vi "DPIDs.CompileServices.vi"(8 "error in (no error)":errorcluster, 11 "Section Ref in":T6 format="%.0x") -> (0 "error out":errorcluster, 1 "DPIDs Settings":T1[](array[typedef]), 2 "Settings":T3 {"Signal.Cmd.Refs"."Signal Refs" format="%.0x"; "Signal.Cmd.Info"."Signals"."Byte Order" items=["Little Endian", "Big Endian"]; "Signal.Cmd.Info"."Signals"."Data Type" items=["Signed", "Unsigned", "IEEE Float"]; "Settings.Refs"."Signal Refs" format="%.0x"; "Signal.Resp.Refs"."Signal Refs" format="%.0x"; "Signal.Resp.Info"."Signals"."Byte Order" items=["Little Endian", "Big Endian"]; "Signal.Resp.Info"."Signals"."Data Type" items=["Signed", "Unsigned", "IEEE Float"]; "Trigger.Refs"."Signal Refs" format="%.0x"; "Status.Refs"."Signal Refs" format="%.0x"}, 3 "Section Ref out":T6 format="%.0x")   [LabVIEW 2019, in "Diagnostics Addon System Explorer.lvlib"]
uses:
  Diagnostics Addon System Explorer.lvlib
  <vilib>/NI VeriStand/Custom Device API/Custom Device Item Ref.ctl
  Types/Service.Export.ctl
  Types/Frame.Ref.ctl
  Shared/Types/Type.ctl
  Shared/Types/Frame.Compile.ctl
  Shared/Types/Signal.ctl
  Shared/Types/DPID.ctl
  Shared/Types/DPID.Rate.ctl
  Types/FG.Action.ctl
  ID.FG.vi
  Shared/SubVIs/Constants.vi
  <vilib>/NI VeriStand/Custom Device Tools/Custom Device Utility Library/NI VeriStand - Search for All Items by GUID.vi
  <vilib>/NI VeriStand/Custom Device Tools/Custom Device Utility Library/NI VeriStand - Search for Item by GUID.vi
  <vilib>/NI VeriStand/Custom Device API/NI VeriStand - Get Item Children.vi
  <vilib>/NI VeriStand/Custom Device Tools/Custom Device Utility Library/NI VeriStand - Search for Item by Name.vi
  <vilib>/NI/NI VeriStand Advanced SysDef API/SysDef API/SysDef.Property.Set.vi
  <vilib>/NI/NI VeriStand Advanced SysDef API/_SubVIs/SysDef.Property.Set.U32.vi
  <vilib>/NI VeriStand/Custom Device API/NI VeriStand - Get Item Property.vi
  <vilib>/NI VeriStand/Custom Device API/Get Item Property (U32).vi
  <vilib>/NI/NI VeriStand Advanced SysDef API/_SubVIs/SysDef.Property.Set.U32.Array.vi
  <vilib>/NI VeriStand/Custom Device API/Get Item Property (U32 Array).vi
  <vilib>/NI VeriStand/Custom Device Tools/Custom Device Utility Library/Custom Device Utility Library.lvlib
  <vilib>/NI VeriStand/Custom Device API/Custom Device API.lvlib
  Shared/Diagnostics Addon Shared.lvlib
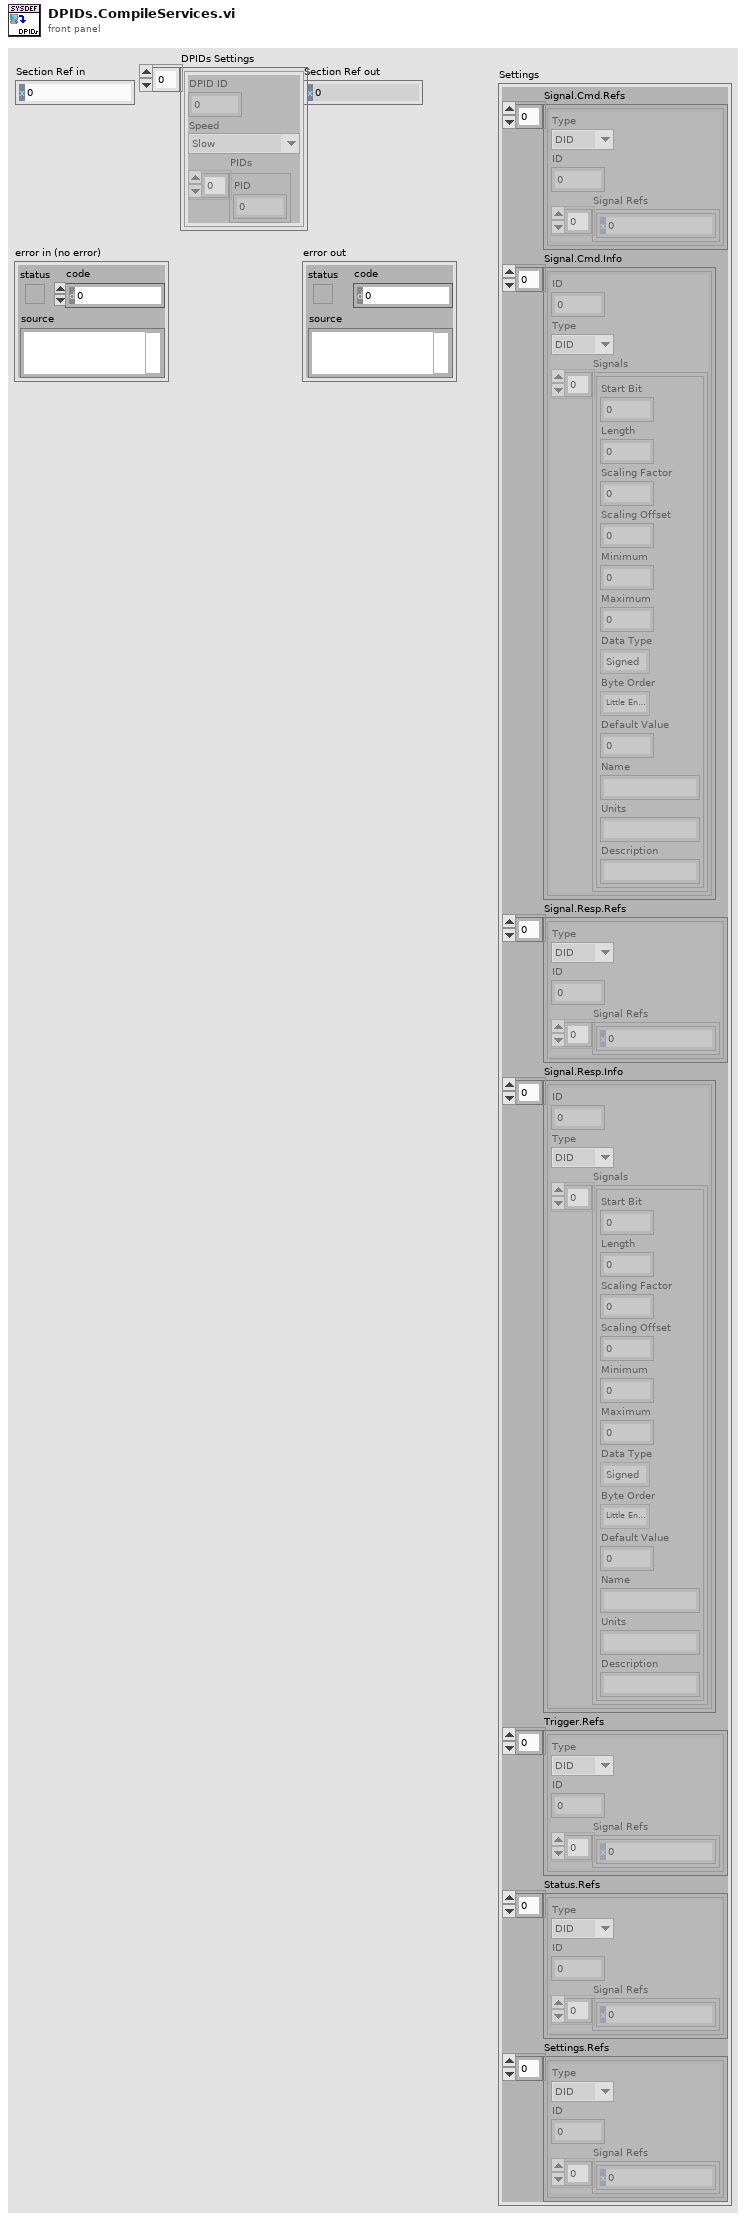
[diagram p1: front panel]
types:
  T1 = typedef "Diagnostics Addon Shared.lvlib/DPID.ctl" = cluster{"DPID ID":u8, "Speed":T2, "PIDs":u16[]}
  T2 = typedef "Diagnostics Addon Shared.lvlib/DPID.Rate.ctl" = enum16{"Slow", "Medium", "Fast"}
  T3 = typedef "Diagnostics Addon System Explorer.lvlib/Service.Export.ctl" = cluster{"Signal.Cmd.Refs":T4[], "Signal.Cmd.Info":T7[], "Signal.Resp.Refs":T4[], "Signal.Resp.Info":T7[], "Trigger.Refs":T4[], "Status.Refs":T4[], "Settings.Refs":T4[]}
  T4 = typedef "Diagnostics Addon System Explorer.lvlib/Frame.Ref.ctl" = cluster{"Type":T5, "ID":u32, "Signal Refs":T6[]}
  T5 = typedef "Diagnostics Addon Shared.lvlib/Type.ctl" = enum16{"DID", "CDID", "PID", "CPID", "Read Memory", "Write Memory", "IO Control", "Routine Start", "Routine Request", "Routine Stop", "User Defined", "DTC Control", "Clear DTCs", "Read DTCs", "Start DTCs", "DTC Change Count", "Tester Present", "Unlock ECU", "Reset ECU", "Diag Session Control", "Communication Control", "DPID Control", "Poll Control", "Diag CAN Control"}
  T6 = typedef "Custom Device API.lvlib/Custom Device Item Ref.ctl" = u64
  T7 = typedef "Diagnostics Addon Shared.lvlib/Frame.Compile.ctl" = cluster{"ID":u32, "Type":T5, "Signals":T8[]}
  T8 = typedef "Diagnostics Addon Shared.lvlib/Signal.ctl" = cluster{"Start Bit":u32, "Length":u32, "Scaling Factor":dbl, "Scaling Offset":dbl, "Minimum":dbl, "Maximum":dbl, "Data Type":u32, "Byte Order":u32, "Default Value":dbl, "Name":string, "Units":string, "Description":string}
  T9 = typedef "Diagnostics Addon System Explorer.lvlib/FG.Action.ctl" = enum16{"Get", "Set"}
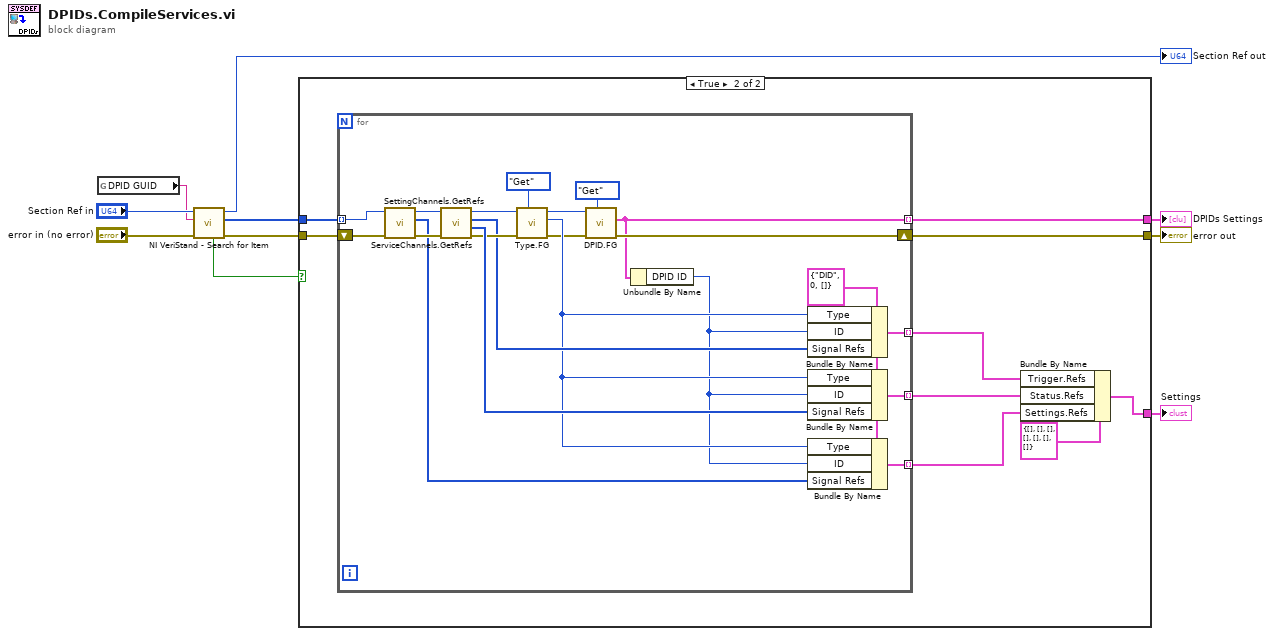
[diagram p0: block diagram]
diagram:
  n1 = global read "Constants.vi" "DPID GUID"() -> (w2:string)
  n2 = call-poly <vilib>:"NI VeriStand - Search for Item.vi"("error in"="error in (no error)", "Item GUID"=w2, "Section Ref in"="Section Ref in") -> ("error out"=w5:errorcluster, "Item Refs"=w6:T6[], "Section Ref out"=→"Section Ref out":T6, "Found"=w4:bool)  [unwired: 5 in]
  n3 = case shown="True" w4 {
    tunnel: [w11 w20] -> w9
    tunnel: w6 -> [_ w13]
    tunnel: w5 -> [w11 w14]
    tunnel: [_ w16] -> w3
    tunnel: [_ w12] -> w1
    frame False {
    }
    frame True {
      n4 = for {
        shift-right: [w25] -> w20
        shift-left: w14 -> [w35]
        tunnel: w13 -> [w32] mode=indexing
        tunnel: [w36] -> w19 mode=indexing
        tunnel: [w31] -> w18 mode=indexing
        tunnel: [w27] -> w15 mode=indexing
        tunnel: [w21] -> w12 mode=indexing
        w30 = T4 {"Type"=enum."DID", "ID"=0, "Signal Refs"=[]} ("cluster")
        n5 = call "SettingChannels.GetRefs.vi"("error in (no error)"=w35, "Item Ref in"=w32) -> ("error out"=w34:errorcluster, "Settings"=w29:T6[], "Section Ref out"=w33:T6)  [unwired: 7 in]
        n6 = call "ServiceChannels.GetRefs.vi"("error in (no error)"=w34, "Item Ref in"=w33) -> ("error out"=w38:errorcluster, "Status"=w39:T6[], "Trigger"=w37:T6[], "Section Ref out"=w40:T6)  [unwired: 6 in]
        n7 = call "Type.FG.vi"("Action"=FG.Action."Get", "error in (no error)"=w38, "Device Item Ref in"=w40) -> ("error out"=w22:errorcluster, "Type"=w28:T5, "Device Item Ref out"=w23:T6)  [unwired: 6 in]
        n8 = call "DPID.FG.vi"("Action"=FG.Action."Get", "error in (no error)"=w22, "Device Item Ref in"=w23) -> ("error out"=w25:errorcluster, "DPID"=w21:T1)  [unwired: 6 in, 1 out]
        n9 = Unbundle By Name(w21) -> ("DPID ID"=w24:u8)
        n10 = Bundle By Name(cluster=w30, "Type"=w28, "ID"=w24, "Signal Refs"=w37) -> (w36:T4)
        n11 = Bundle By Name(cluster=w30, "Type"=w28, "ID"=w24, "Signal Refs"=w39) -> (w31:T4)
        n12 = Bundle By Name(cluster=w30, "Type"=w28, "ID"=w24, "Signal Refs"=w29) -> (w27:T4)
      }
      n13 = Bundle By Name(cluster=T3 {"Signal.Cmd.Refs"=[], "Signal.Cmd.Info"=[], "Signal.Resp.Refs"=[], "Signal.Resp.Info"=[], "Trigger.Refs"=[], "Status.Refs"=[], "Settings.Refs"=[]}, "Trigger.Refs"=w19, "Status.Refs"=w18, "Settings.Refs"=w15) -> (w16:T3)
    }
  }
  "error out" <- w9
  "Settings" <- w3
  "DPIDs Settings" <- w1
